vi "get Broadcast Ping Result.vi"(9 "id":i32, 10 "protocol_version":i32, 11 "port_num":i32) -> (3 "function return":u8)   [LabVIEW 2016, in "dxl_x86_c.lvlib"]
doc: "WINDECLSPEC uint8_t getBroadcastPingResult (int port_num, int protocol_version, int id);"
uses:
  dxl_x86_c.lvlib
  dxl_x86_c.dll
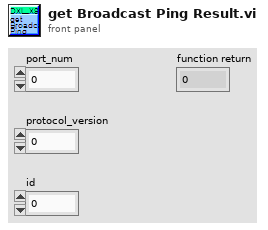
[diagram p1: front panel]
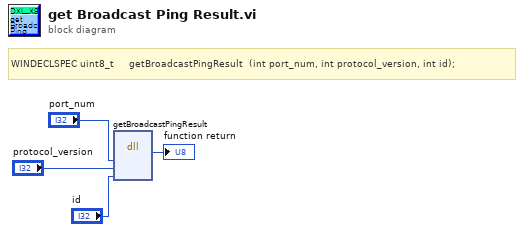
[diagram p0: block diagram]
diagram:
  # "WINDECLSPEC uint8_t     getBroadcastPingResult  (int port_num, int protocol_version, int id);"
  n1 = dll-call lib="C:/Users/Platform/Desktop/GITHUB/DynamixelSDK/labview/dxl_x86_c.lvlib/dxl_x86_c.*" fn="getBroadcastPingResult"("port_num"="port_num", "protocol_version"="protocol_version", "id"="id") -> (→"function return":u8)  [unwired: 6 in, 2 out]
